vi "Init Grove I2C Switch.vi"(8 "error in (no error)":errorcluster, 10 "Address":u8=17 caption="(Default x11)" format="%.0x", 11 "I2C RGB SGM31323 in":refnum<class "4ChannelSPDTRelay.lvclass">) -> (0 "error out":errorcluster, 3 "I2C RGB SGM31323 out":refnum<class "4ChannelSPDTRelay.lvclass">)   [LabVIEW 2020, in "CTI-Peripheral.lvlib" / "4ChannelSPDTRelay.lvclass"]
uses:
  4ChannelSPDTRelay.lvclass
  4ChannelSPDTRelay.lvclass/4ChannelSPDTRelay.ctl
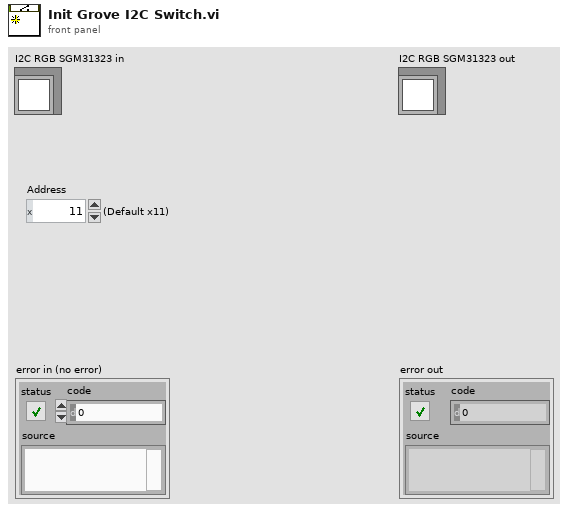
[diagram p1: front panel]
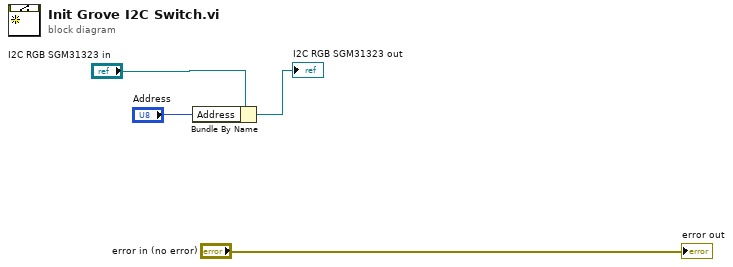
[diagram p0: block diagram]
diagram:
  n1 = Bundle By Name(cluster="I2C RGB SGM31323 in", "Address"="Address") -> (→"I2C RGB SGM31323 out":refnum<class "4ChannelSPDTRelay.lvclass">)
  "error out" <- "error in (no error)"
